vi "Select Log File.vi"(11 "Error IN":errorcluster) -> (4 "Log File OUT":path, 15 "Error OUT":errorcluster)   [LabVIEW 2011]
uses:
  Data Manager/Controls/Path.ctl
panel:
  in  "Continue":bool
  in  "Cancel Button":bool
  in  "Select Log File":T1
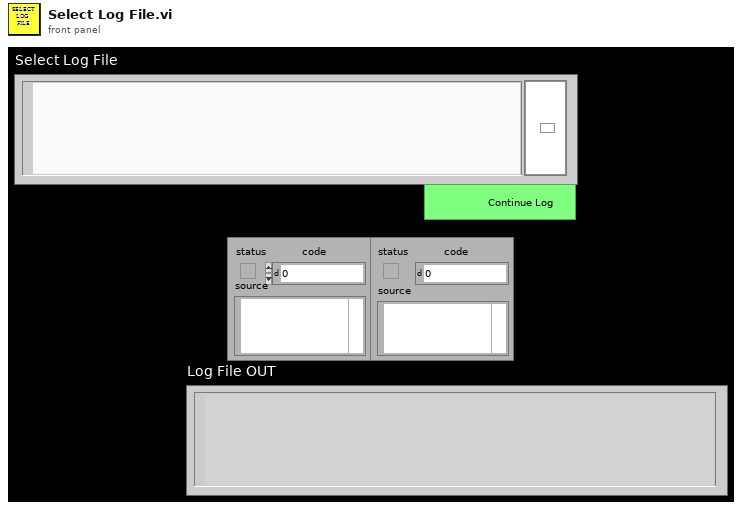
[diagram p1: front panel]
types:
  T1 = typedef "Path.ctl" = path
  T2 = enum16{"open", "replace", "create", "open or create", "replace or create", "replace or create with confirmation"}
  T3 = cluster{"Main Panel Path":path, "Config Directory":path, "Log Directory":path}
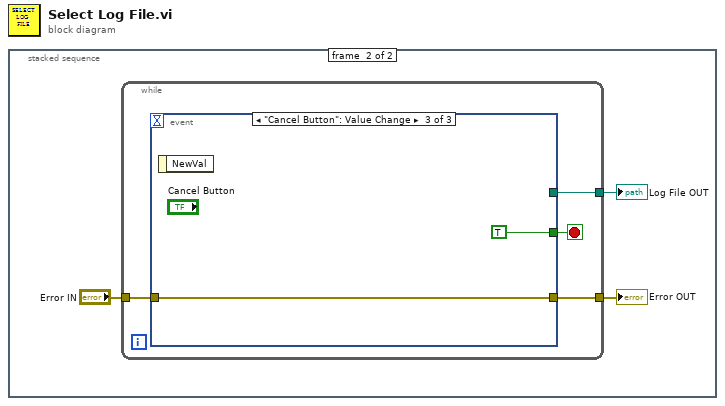
[diagram p0: block diagram]
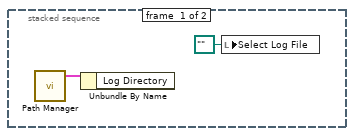
[diagram p2: hidden frame]
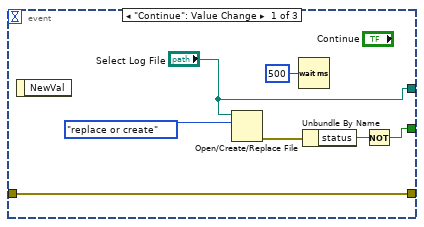
[diagram p3: hidden frame]
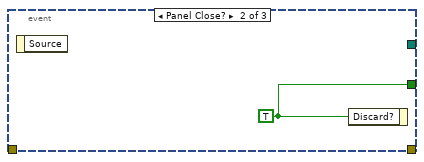
[diagram p4: hidden frame]
diagram:
  n1 = stacked-sequence {
    frame #0 {
      n2 = call "Path Manager.vi"() -> ("Path Location Cluster"=w2:T3)  [unwired: 14 in, 1 out]
      n3 = Unbundle By Name(w2) -> ()  [unwired: 1 out]
      n4 = local write "Select Log File"(path "" ("Select Log File")) -> ()
    }
    frame #1 {
      n5 = while {
        tunnel: "Error IN" -> [w9]
        tunnel: [w8] -> w4
        tunnel: [w6] -> w3
        stop <- w7 stop-if-true
        n6 = event shown="[2] \"Cancel Button\": Value Change" {
          selector: _ -> [_ _ _]
          dyn-events: _ -> [_ _ _]
          timeout: _ -> [_ _ _]
          tunnel: [w16 _ w19] -> w8
          tunnel: w9 -> [w16 _ w19]
          tunnel: [w10 w17 TRUE] -> w7
          tunnel: ["Select Log File" _ _] -> w6
          event "Continue": Value Change {
            n7 = event-data() -> ()  [unwired: 1 in, 1 out]
            n8 = Open/Create/Replace File(file path (use dialog)="Select Log File", operation (0:open)=T2."replace or create") -> (error out=w12:errorcluster)  [unwired: 4 in, 2 out]
            n9 = Wait (ms)(milliseconds to wait=u32 500) -> ()  [unwired: 1 out]
            n10 = Unbundle By Name(w12) -> ("status"=w11:bool)
            n11 = Not(x=w11) -> (.not. x?=w10:bool)
          }
          event Panel Close? {
            w17 = TRUE ("Discard?")
            n12 = event-data() -> ()  [unwired: 1 in, 1 out]
            n13 = event-data("Discard?"=w17) -> ()  [unwired: 1 in, 1 out]
          }
          event "Cancel Button": Value Change {
            n14 = event-data() -> ()  [unwired: 1 in, 1 out]
          }
        }
      }
      "Error OUT" <- w4
      "Log File OUT" <- w3
    }
  }
